vi "compare_arrays.vi"(1 "Array - Numeric 2":dbl[](array[numeric]), 2 "Array - Numeric":dbl[](array[numeric])) -> (0 "Numeric Control":dbl)   [LabVIEW 2015]
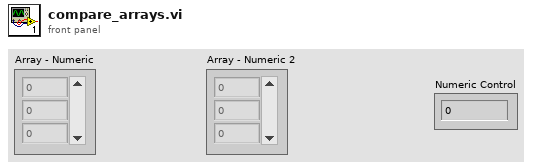
[diagram p1: front panel]
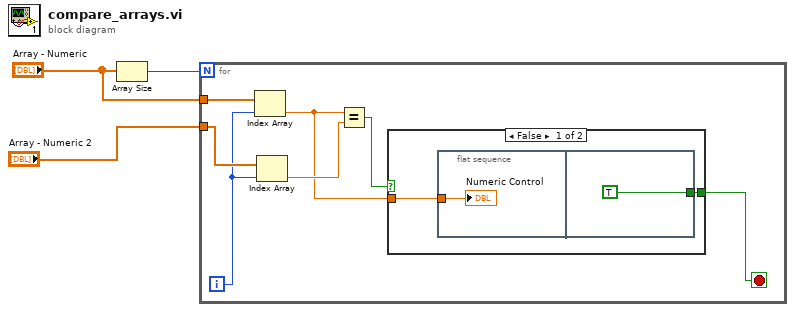
[diagram p0: block diagram]
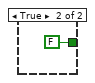
[diagram p2: hidden frame]
diagram:
  n1 = Array Size(array="Array - Numeric") -> (size(s)=w3:i32)
  n2 = for {
    N: w3 -> [_]
    tunnel: "Array - Numeric" -> [w10]
    tunnel: "Array - Numeric 2" -> [w9]
    i -> [w8]
    stop <- w4 stop-if-true
    n3 = Index Array(array=w10, index=w8) -> (element=w5:dbl)
    n4 = Index Array(array=w9, index=w8) -> (element=w7:dbl)
    n5 = Equal?(x=w5, y=w7) -> (x = y?=w6:bool)
    n6 = case shown="False" w6 {
      tunnel: w5 -> [w12 _]
      tunnel: [w11 FALSE] -> w4
      frame False {
        n7 = flat-sequence {
          tunnel: w12 -> [w13]
          tunnel: [TRUE] -> w11
          frame #0 {
            "Numeric Control" <- w13
          }
          frame #1 {
          }
        }
      }
      frame True {
      }
    }
  }
